vi "Grab Record String.vi"(9 "Raw Binary String":string, 11 "Offset":i32) -> (1 "Record String":string, 3 "New Offset":i32)   [LabVIEW 2019, in "ParseGDSII.lvclass"]
uses:
  ParseGDSII.lvclass
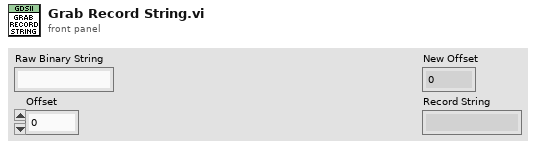
[diagram p1: front panel]
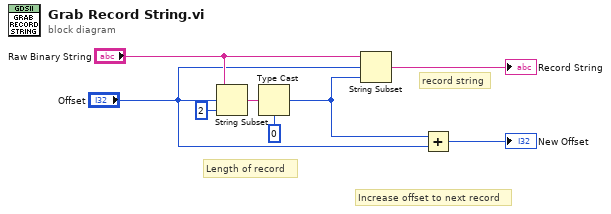
[diagram p0: block diagram]
diagram:
  # "record string"
  # "Increase offset to next record"
  # "Length of record"
  n1 = String Subset(string="Raw Binary String", offset (0)="Offset", length (rest)=2 ("length (rest)")) -> (substring=w7:string)
  n2 = Type Cast(type=i16 0, x=w7) -> (*(type *) &x=w2:i16)
  n3 = String Subset(string="Raw Binary String", offset (0)="Offset", length (rest)=w2) -> (substring=→"Record String":string)
  n4 = Add(x=w2, y="Offset") -> (x+y=→"New Offset":i32)
